vi "Format Variant Into String--EasyXML.vi"(0 "Input String":string, 2 "format string":string, 7 "error in (no error)":errorcluster, 11 "Variant":variant) -> (4 "Output String":string, 8 "error out":errorcluster)   [LabVIEW 2013]
doc: "Overcomes a limitation of \"Format Into String\" by allowing variant data types to be used. This VI supports variant data for all LabVIEW data types supported by \"Format Into String\". The \"format string\" input may optionally be passed as an variant attribute named \"Format String\"."
uses:
  JKI Reuse Candidates/Is an Error (error cluster)__JKI Error Handling.vi
panel:
  # "[OpenG VI Tags] ***Do Not Remove***\nSVN Revision = 386\nSVN Revision Date = 2006-11-25 12:03:42 -0800 (Sat, 25 Nov 2006)\nPackage = oglib_string-2.6-1\nDepends ="
  # "JK 2007-11-11: Added support for timestamp and enum %d format strings"
  # "Format Variant Into String.vi\n\nOvercomes a limitation of \"Format Into String\" by allowing variant data types to be used.  This VI supports variant data for all LabVIEW data types supported by\n\"Format Into String\".  The \"format string\" input may optionally be passed as an variant attribute named \"Format String\"\n\nPlease visit http://www.OpenG.org to learn about the\nOpen Source LabVIEW software movement.\n\nNOTICE -- YOU MUST LEAVE THIS NOTICE IN PLACE.  PER THE TERMS OF THE LICENSE BELOW, YOU MAY SUBLICENSE THIS SOFTWARE \nIN ANY WAY THAT DOES NOT CONFLICT WITH THIS LICENSE.\n\n### BSD License (http://www.opensource.org/licenses/bsd-license.php) Begin ###\n \nCopyright (c) 2002-2004, Jim Kring <jim@jimkring.com>\nCopyright (c) 2004, Michael C. Ashe <michael.ashe@imaginatics.com>\n\nAll rights reserved.\n\nRedistribution and use in source and binary forms, with or without modification, are permitted provided that the following conditions are met:\n\n    * Redistributions of source code must retain the above copyright notice, this list of conditions and the following disclaimer.\n    * Redistributions in binary form must reproduce the above copyright notice, this list of conditions and the following disclaimer in the \n       documentation and/or other materials provided with the distribution.\n    * Neither the name of SciWare, James Kring, Inc., nor the names of its contributors may be used to endorse or promote products derived \n       from this software without specific prior written permission.\n\nTHIS SOFTWARE IS PROVIDED BY THE COPYRIGHT HOLDERS AND CONTRIBUTORS \"AS IS\" AND ANY EXPRESS OR IMPLIED WARRANTIES, \nINCLUDING, BUT NOT LIMITED TO, THE IMPLIED WARRANTIES OF MERCHANTABILITY AND FITNESS FOR A PARTICULAR PURPOSE ARE \nDISCLAIMED. IN NO EVENT SHALL THE COPYRIGHT OWNER OR CONTRIBUTORS BE LIABLE FOR ANY DIRECT, INDIRECT, INCIDENTAL,\n SPECIAL, EXEMPLARY, OR CONSEQUENTIAL DAMAGES (INCLUDING, BUT NOT LIMITED TO, PROCUREMENT OF SUBSTITUTE GOODS OR \nSERVICES; LOSS OF USE, DATA, OR PROFITS; OR BUSINESS INTERRUPTION) HOWEVER CAUSED AND ON ANY THEORY OF LIABILITY, \nWHETHER IN CONTRACT, STRICT LIABILITY, OR TORT (INCLUDING NEGLIGENCE OR OTHERWISE) ARISING IN ANY WAY OUT OF THE USE \nOF THIS SOFTWARE, EVEN IF ADVISED OF THE POSSIBILITY OF SUCH DAMAGE.\n\n### BSD License End ###"
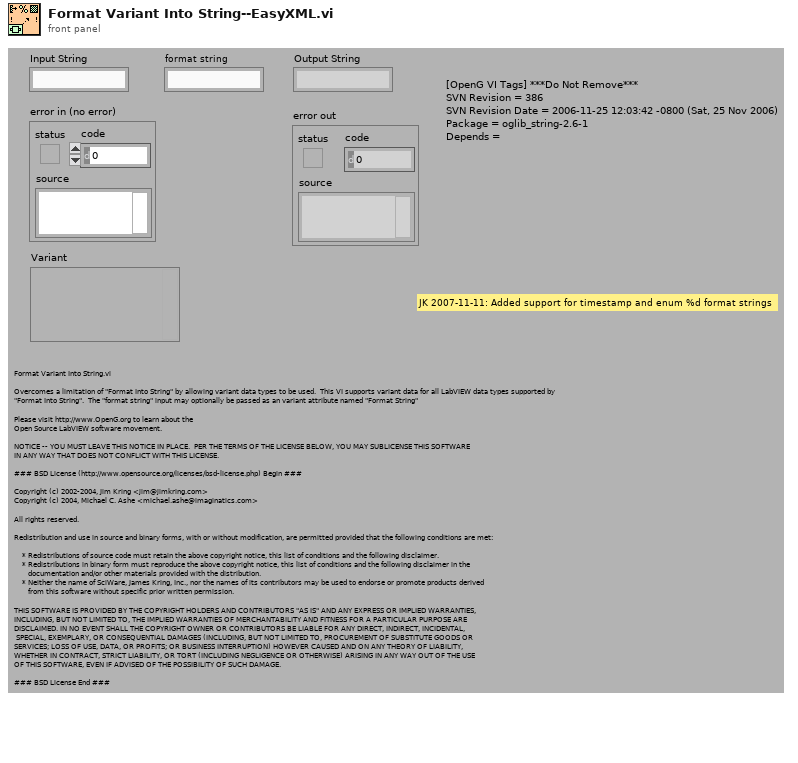
[diagram p1: front panel]
types:
  T1 = typedef "Type Descriptor Enumeration__ogtk.ctl" = enum8{"<Null>", "I8", "I16", "I32", "I64", "U8", "U16", "U32", "U64", "SGL", "DBL", "EXT", "CSG", "CDB", "CXT", "0x0F", "0x10", "0x11", "0x12", "0x13", "0x14", "Enum U8", "Enum U16", "Enum U32", "Enum U64", "SGL PQ", "DBL PQ", "EXT PQ", "CSG PQ", "CDB PQ", "CXT PQ", "0x1F", "0x20", "Boolean", "0x22", "0x23", "0x24", "0x25", "0x26", "0x27", "0x28", "0x29", "0x2A", "0x2B", "0x2C", "0x2D", "0x2E", "0x2F", "String", "0x31", "Path", "Pict", "0x34", "0x35", "0x36", "DAQ", "0x38", "0x39", "0x3A", "0x3B", "0x3C", "0x3D", "0x3E", "0x3F", "Array", "0x41", "0x42", "0x43", "0x44", "0x45", "0x46", "0x47", "0x48", "0x49", "0x4A", "0x4B", "0x4C", "0x4D", "0x4E", "0x4F", "Cluster", "0x51", "0x52", "Variant", "Waveform", "0x55", "0x56", "0x57", "0x58", "0x59", "0x5A", "0x5B", "0x5C", "0x5D", "0x5E", "0x5F", "0x60", "0x61", "0x62", "0x63", "0x64", "0x65", "0x66", "0x67", "0x68", "0x69", "0x6A", "0x6B", "0x6C", "0x6D", "0x6E", "0x6F", "Refnum"}
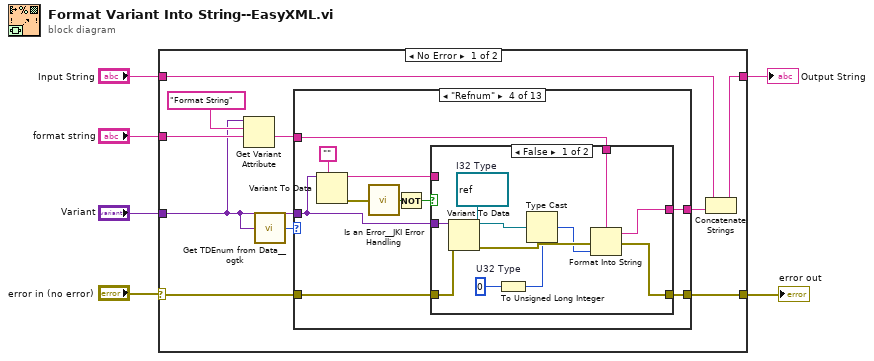
[diagram p0: block diagram]
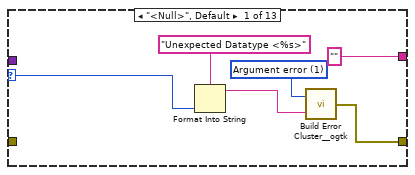
[diagram p2: hidden frame]
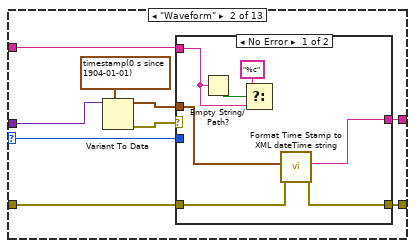
[diagram p3: hidden frame]
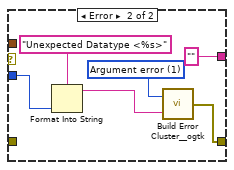
[diagram p4: hidden frame]
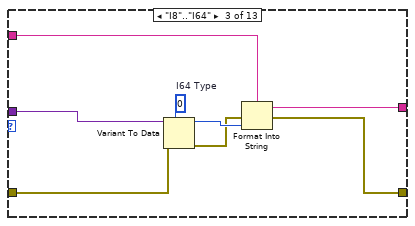
[diagram p5: hidden frame]
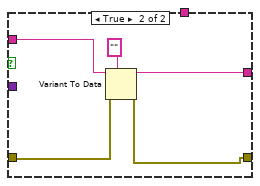
[diagram p6: hidden frame]
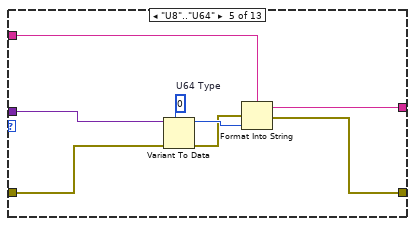
[diagram p7: hidden frame]
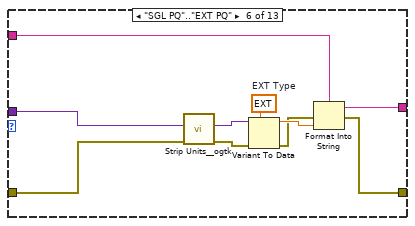
[diagram p8: hidden frame]
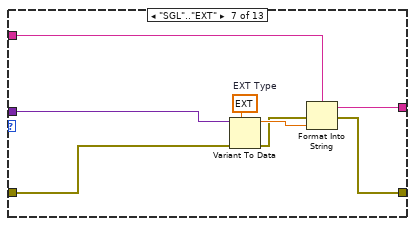
[diagram p9: hidden frame]
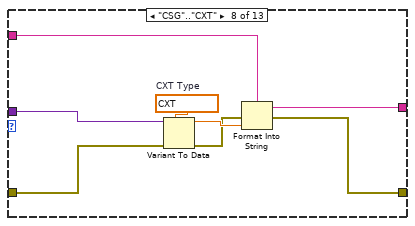
[diagram p10: hidden frame]
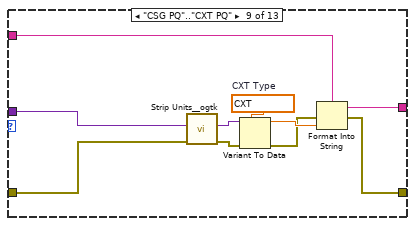
[diagram p11: hidden frame]
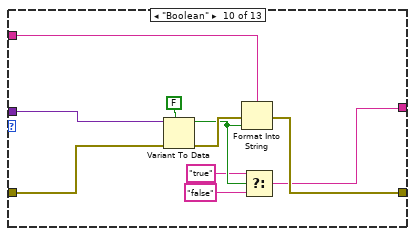
[diagram p12: hidden frame]
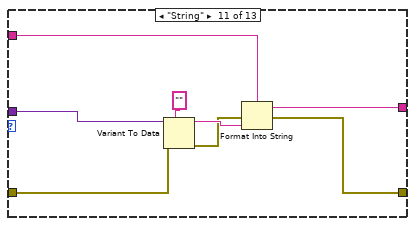
[diagram p13: hidden frame]
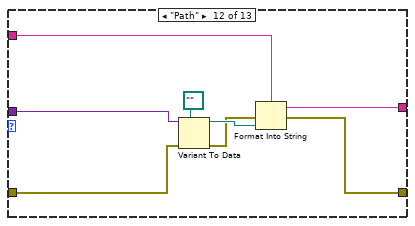
[diagram p14: hidden frame]
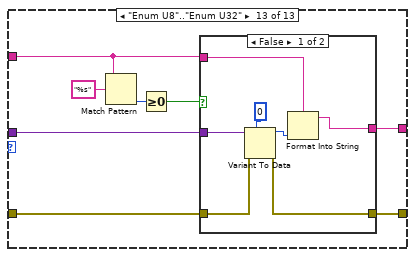
[diagram p15: hidden frame]
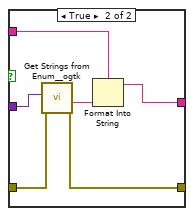
[diagram p16: hidden frame]
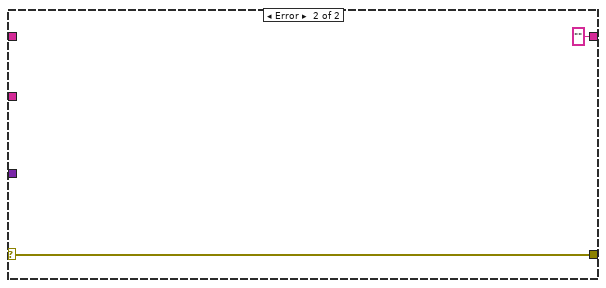
[diagram p17: hidden frame]
diagram:
  n1 = case shown="No Error" "error in (no error)" {
    selector: "error in (no error)" -> [w14 w171]
    tunnel: "Input String" -> [w11 _]
    tunnel: [w15 ""] -> w5
    tunnel: "format string" -> [w10 _]
    tunnel: "Variant" -> [w8 _]
    tunnel: [w13 w171] -> w1
    frame No Error {
      n2 = Get Variant Attribute(Variant=w8, name="Format String", default value (empty Variant)=w10) -> (value=w9:string)  [unwired: 1 in, 3 out]
      n3 = call <userlib>:"Get TDEnum from Data__ogtk.vi"("Data"=w8) -> ("Type Descriptor Enumeration"=w7:T1)  [unwired: 4 in]
      n4 = case shown="\"Refnum\"" w7 {
        selector: w7 -> [w18 w30 _ _ _ _ _ _ _ _ _ _ _]
        tunnel: w8 -> [_ w28 w51 w55 w85 w89 w98 w111 w115 w132 w140 w148 w156]
        tunnel: w9 -> [_ w24 w49 w62 w83 w94 w102 w109 w120 w127 w138 w146 w149]
        tunnel: ["" w31 w48 w61 w82 w93 w101 w108 w119 w123 w137 w145 w154] -> w16
        tunnel: [w17 w29 w45 w59 w79 w91 w99 w105 w117 w128 w134 w141 w153] -> w13
        tunnel: w14 -> [_ w23 w47 w60 w81 w88 w97 w107 w114 w130 w133 w143 w155]
        frame "<Null>", Default {
          w21 = 1 items=["No error", "Argument error", "Memory is full", "Out of zone", "End of file", "File already open", "Generic file I/O error", "File not found", "File permission error", "Disk is full", "Duplicate path", "Too many files open", "System feature not enabled", "Resource file not found", "Cannot add resource", "Resource not found", "Image not found", "Image memory error", "Pen does not exist", "Config type invalid", "Config token not found", "Config parse error", "Config memory error", "Bad external code format", "Bad external code offset", "External code not present", "Null window", "Destroy window error", "Null menu", "Print aborted", "Bad print record", "Print driver error", "Windows error during printing", "Memory error during printing", "Print dialog error", "Generic print error", "Invalid device refnum", "Device not found", "Device parameter error", "Device unit error", "Cannot open device", "Device call aborted", "Generic error", "Cancelled by user", "Object ID too low", "Object ID too high", "Object not in heap", "Unknown heap", "Unknown object (invalid DefProc)", "Unknown object (DefProc not in table)", "Message out of range", "Invalid (null) method", "Unknown message", "Manager call not supported", "Bad address", "Network operation in progress", "Network operation timed out", "Connection is busy", "Network attribute not supported", "Network error", "Address in use", "System out of memory", "Connection aborted", "Connection refused", "Not connected", "Already connected", "Connection closed", "Initialization error (interapplication manager)", "Bad occurrence", "Wait on unbound occurrence handler", "Occurrence queue overflow", "Datalog type conflict", "Unused", "Unrecognized type (interapplication manager)", "Memory corrupt", "Failed to make temporary DLL", "Old CIN version", "Drag socket not found", "Failed to load drop-object", "Failed to register OLE object", "Failed to release OLE object", "Format specifier type mismatch", "Unknown format specifier", "Too few format specifiers", "Too many format specifiers", "Scan failed", "Newer CIN version", "Error converting to variant", "Runtime menu error", "Password tampered", "Variant attribute not found", "Incompatible variant data type", "Event data is not available", "Event Store is not present", "Occurrence is not found", "Event Queue is not created", "Event info is not available", "Refnum passed is NULL", "Error retrieving Class GUID", "Error retrieving CoClass GUID", "Error retrieving TypeLib GUID.", "Bad built application magic bytes.", "Specific driver is different from the specific driver associated with the Logical Name.", "There is no session opened to the class driver.", "Max Error", "MAX - Error with config objects", "MAX - Error loading configuration", "MAX - Group not supported"]
          n5 = Format Into String(format string="Unexpected Datatype <%s>" ("Format String"), w18) -> (resulting string=w19:string)  [unwired: 2 in, 1 out]
          n6 = call <userlib>:"Build Error Cluster__ogtk.vi"("String to Prepend to source (\"\")"=w19, "code"=w21) -> ("error out"=w17:errorcluster)
        }
        frame "Waveform" {
          n7 = Variant To Data(type=timestamp(0 s since 1904-01-01), Variant=w28) -> (data=w25:timestamp, error out=w26:errorcluster)  [unwired: 1 in]
          n8 = case shown="No Error" w26 {
            tunnel: [w34 ""] -> w31
            tunnel: w30 -> [_ w40]
            tunnel: [w32 w39] -> w29
            tunnel: w25 -> [w35 _]
            tunnel: w24 -> [w37 _]
            tunnel: w23 -> [w33 _]
            frame No Error {
              n9 = Empty String/Path?(string/path=w37) -> (empty?=w38:bool)
              n10 = Select(t="%c", s=w38, f=w37) -> ()  [unwired: 1 out]
              n11 = call "Format Time Stamp to XML dateTime string.vi"("error in (no error)"=w33, "time stamp"=w35) -> ("error out"=w32:errorcluster, "xml dateTime string"=w34:string)  [unwired: 8 in]
            }
            frame Error {
              w43 = 1 items=["No error", "Argument error", "Memory is full", "Out of zone", "End of file", "File already open", "Generic file I/O error", "File not found", "File permission error", "Disk is full", "Duplicate path", "Too many files open", "System feature not enabled", "Resource file not found", "Cannot add resource", "Resource not found", "Image not found", "Image memory error", "Pen does not exist", "Config type invalid", "Config token not found", "Config parse error", "Config memory error", "Bad external code format", "Bad external code offset", "External code not present", "Null window", "Destroy window error", "Null menu", "Print aborted", "Bad print record", "Print driver error", "Windows error during printing", "Memory error during printing", "Print dialog error", "Generic print error", "Invalid device refnum", "Device not found", "Device parameter error", "Device unit error", "Cannot open device", "Device call aborted", "Generic error", "Cancelled by user", "Object ID too low", "Object ID too high", "Object not in heap", "Unknown heap", "Unknown object (invalid DefProc)", "Unknown object (DefProc not in table)", "Message out of range", "Invalid (null) method", "Unknown message", "Manager call not supported", "Bad address", "Network operation in progress", "Network operation timed out", "Connection is busy", "Network attribute not supported", "Network error", "Address in use", "System out of memory", "Connection aborted", "Connection refused", "Not connected", "Already connected", "Connection closed", "Initialization error (interapplication manager)", "Bad occurrence", "Wait on unbound occurrence handler", "Occurrence queue overflow", "Datalog type conflict", "Unused", "Unrecognized type (interapplication manager)", "Memory corrupt", "Failed to make temporary DLL", "Old CIN version", "Drag socket not found", "Failed to load drop-object", "Failed to register OLE object", "Failed to release OLE object", "Format specifier type mismatch", "Unknown format specifier", "Too few format specifiers", "Too many format specifiers", "Scan failed", "Newer CIN version", "Error converting to variant", "Runtime menu error", "Password tampered", "Variant attribute not found", "Incompatible variant data type", "Event data is not available", "Event Store is not present", "Occurrence is not found", "Event Queue is not created", "Event info is not available", "Refnum passed is NULL", "Error retrieving Class GUID", "Error retrieving CoClass GUID", "Error retrieving TypeLib GUID.", "Bad built application magic bytes.", "Specific driver is different from the specific driver associated with the Logical Name.", "There is no session opened to the class driver.", "Max Error", "MAX - Error with config objects", "MAX - Error loading configuration", "MAX - Group not supported"]
              n12 = Format Into String(format string="Unexpected Datatype <%s>" ("Format String"), w40) -> (resulting string=w41:string)  [unwired: 2 in, 1 out]
              n13 = call <userlib>:"Build Error Cluster__ogtk.vi"("String to Prepend to source (\"\")"=w41, "code"=w43) -> ("error out"=w39:errorcluster)
            }
          }
        }
        frame "I8".."I64" {
          w52 = i64 0  # I64 Type
          n14 = Variant To Data(error in=w47, type=w52, Variant=w51) -> (data=w50:i64, error out=w46:errorcluster)
          n15 = Format Into String(format string=w49, error in=w46, w50) -> (resulting string=w48:string, error out=w45:errorcluster)  [unwired: 1 in]
        }
        frame "Refnum" {
          n16 = Variant To Data(type="", Variant=w55) -> (data=w53:string, error out=w56:errorcluster)  [unwired: 1 in]
          n17 = call-poly "Is an Error__JKI Error Handling.vi"("error in"=w56) -> ("error?"=w57:bool)  [unwired: 8 in]
          n18 = Not(x=w57) -> (.not. x?=w54:bool)
          n19 = case shown="False" w54 {
            tunnel: w62 -> [w71 _]
            tunnel: [w70 w76] -> w61
            tunnel: w60 -> [w69 w74]
            tunnel: [w67 w75] -> w59
            tunnel: w55 -> [w63 _]
            tunnel: w53 -> [_ w78]
            frame False {
              w65 = u32 0  # U32 Type
              w73 = refnum<k0> refnum  # I32 Type
              n20 = Variant To Data(error in=w69, type=w73, Variant=w63) -> (data=w72:refnum<k0>, error out=w68:errorcluster)
              n21 = To Unsigned Long Integer(number=w65) -> (unsigned 32bit integer=w64:u32)
              n22 = Type Cast(type=w64, x=w72) -> (*(type *) &x=w66:u32)
              n23 = Format Into String(format string=w71, error in=w68, w66) -> (resulting string=w70:string, error out=w67:errorcluster)  [unwired: 1 in]
            }
            frame True {
              n24 = Variant To Data(error in=w74, type="", Variant=w78) -> (data=w76:string, error out=w75:errorcluster)
            }
          }
        }
        frame "U8".."U64" {
          w86 = u64 0  # U64 Type
          n25 = Variant To Data(error in=w81, type=w86, Variant=w85) -> (data=w84:u64, error out=w80:errorcluster)
          n26 = Format Into String(format string=w83, error in=w80, w84) -> (resulting string=w82:string, error out=w79:errorcluster)  [unwired: 1 in]
        }
        frame "SGL PQ".."EXT PQ" {
          w96 = ext 0.0  # EXT Type
          n27 = call <userlib>:"Strip Units__ogtk.vi"("error in (no error)"=w88, "Number or 1D array with units"=w89) -> ("error out"=w87:errorcluster, "Pure Number(s) (base units)"=w90:variant)  [unwired: 8 in]
          n28 = Variant To Data(error in=w87, type=w96, Variant=w90) -> (data=w95:ext, error out=w92:errorcluster)
          n29 = Format Into String(format string=w94, error in=w92, w95) -> (resulting string=w93:string, error out=w91:errorcluster)  [unwired: 1 in]
        }
        frame "SGL".."EXT" {
          w104 = ext 0.0  # EXT Type
          n30 = Variant To Data(error in=w97, type=w104, Variant=w98) -> (data=w103:ext, error out=w100:errorcluster)
          n31 = Format Into String(format string=w102, error in=w100, w103) -> (resulting string=w101:string, error out=w99:errorcluster)  [unwired: 1 in]
        }
        frame "CSG".."CXT" {
          w112 = cxt 0.0+0.0i  # CXT Type
          n32 = Variant To Data(error in=w107, type=w112, Variant=w111) -> (data=w110:cxt, error out=w106:errorcluster)
          n33 = Format Into String(format string=w109, error in=w106, w110) -> (resulting string=w108:string, error out=w105:errorcluster)  [unwired: 1 in]
        }
        frame "CSG PQ".."CXT PQ" {
          w122 = cxt 0.0+0.0i  # CXT Type
          n34 = call <userlib>:"Strip Units__ogtk.vi"("error in (no error)"=w114, "Number or 1D array with units"=w115) -> ("error out"=w113:errorcluster, "Pure Number(s) (base units)"=w116:variant)  [unwired: 8 in]
          n35 = Variant To Data(error in=w113, type=w122, Variant=w116) -> (data=w121:cxt, error out=w118:errorcluster)
          n36 = Format Into String(format string=w120, error in=w118, w121) -> (resulting string=w119:string, error out=w117:errorcluster)  [unwired: 1 in]
        }
        frame "Boolean" {
          n37 = Variant To Data(error in=w130, type=FALSE, Variant=w132) -> (data=w126:bool, error out=w129:errorcluster)
          n38 = Format Into String(format string=w127, error in=w129, w126) -> (error out=w128:errorcluster)  [unwired: 1 in, 1 out]
          n39 = Select(t="true" ("format string"), s=w126, f="false" ("format string")) -> (s? t:f=w123:string)
        }
        frame "String" {
          n40 = Variant To Data(error in=w133, type="", Variant=w140) -> (data=w139:string, error out=w135:errorcluster)
          n41 = Format Into String(format string=w138, error in=w135, w139) -> (resulting string=w137:string, error out=w134:errorcluster)  [unwired: 1 in]
        }
        frame "Path" {
          n42 = Variant To Data(error in=w143, type=path "", Variant=w148) -> (data=w147:path, error out=w142:errorcluster)
          n43 = Format Into String(format string=w146, error in=w142, w147) -> (resulting string=w145:string, error out=w141:errorcluster)  [unwired: 1 in]
        }
        frame "Enum U8".."Enum U32" {
          n44 = Match Pattern(string=w149, regular expression="%s") -> (offset past match=w151:i32)  [unwired: 1 in, 3 out]
          n45 = Greater Or Equal To 0?(x=w151) -> (x >= 0?=w150:bool)
          n46 = case shown="False" w150 {
            tunnel: w156 -> [w163 w169]
            tunnel: w155 -> [w161 w168]
            tunnel: [w157 w165] -> w154
            tunnel: [w160 w167] -> w153
            tunnel: w149 -> [w158 w164]
            frame False {
              n47 = Variant To Data(error in=w161, type=u32 0, Variant=w163) -> (data=w159:u32, error out=w160:errorcluster)
              n48 = Format Into String(format string=w158, w159) -> (resulting string=w157:string)  [unwired: 2 in, 1 out]
            }
            frame True {
              n49 = call <userlib>:"Get Strings from Enum__ogtk.vi"("error in (no error)"=w168, "Enum"=w169) -> ("error out"=w167:errorcluster, "String Value"=w166:string)  [unwired: 6 in, 2 out]
              n50 = Format Into String(format string=w164, w166) -> (resulting string=w165:string)  [unwired: 2 in, 1 out]
            }
          }
        }
      }
      n51 = Concatenate Strings(w11, w16) -> (w15:string)
    }
    frame Error {
    }
  }
  "Output String" <- w5
  "error out" <- w1
